vi "Lex Text-& UnescapedVariable-Text.vi"(8 "Error In":errorcluster) -> (0 "Error Out":errorcluster)   [LabVIEW 2018, in "Tests.lvlib" / "Lexer.lvlib"]
uses:
  Lexer.lvlib
  <vilib>/addons/_JKI Toolkits/Caraya/classes/Test/Test.lvclass
  <vilib>/addons/_JKI Toolkits/Caraya/classes/Assert/Assert.lvclass
  src/Toolkit/Low-Level/Tokens/Abstract/Abstract.lvclass
  src/Toolkit/Low-Level/Tokens/Text/Text.lvclass
  Tests.lvlib
  src/Toolkit/Low-Level/Tokens/UnescapedVariable/UnescapedVariable.lvclass
  D:/Users/cfield/Code/Field R&D Services/Mustache/trunk/src/Toolkit/Low-Level/Tokens/Abstract/Abstract.lvclass
  src/Toolkit/Toolkit.lvlib
  src/Toolkit/Low-Level/Support/Lex String.vi
  D:/Users/cfield/Code/Field R&D Services/Mustache/trunk/src/Toolkit/Low-Level/Tokens/Keyable/Keyable.lvclass
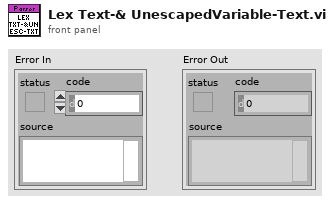
[diagram p1: front panel]
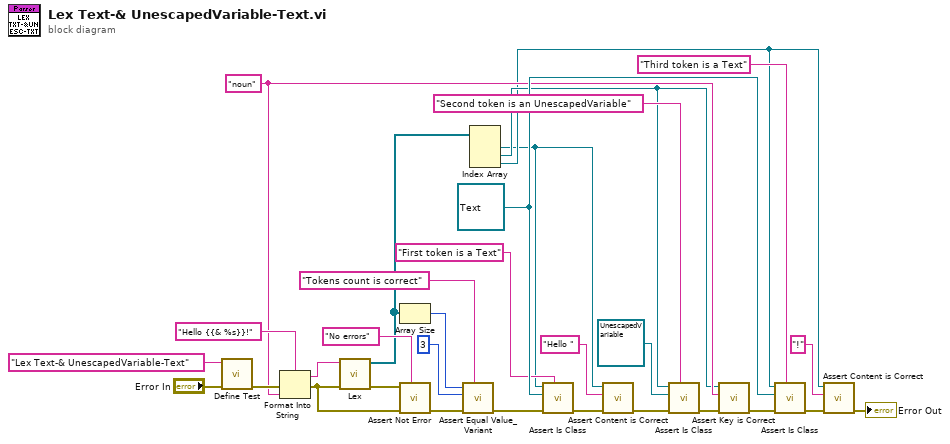
[diagram p0: block diagram]
diagram:
  w13 = refnum<class "Text.lvclass"> refnum ("Mustache.lvlib:Tokens.lvlib:Text.lvclass")
  w9 = "noun" ("String")
  n1 = call <vilib>:"Define Test.vi"("error in (no error)"="Error In", "Label (VI Title)"="Lex Text-& UnescapedVariable-Text") -> ("error out"=w28:errorcluster)  [unwired: 9 in]
  n2 = Format Into String(format string="Hello {{& %s}}!", error in=w28, w9) -> (resulting string=w1:string, error out=w2:errorcluster)  [unwired: 1 in]
  n3 = call-poly "Lex.vi"("Error In"=w2, "Input"=w1) -> ("Error Out"=w29:errorcluster, "Tokens"=w21:refnum<class "Abstract.lvclass">[])  [unwired: 8 in]
  n4 = Array Size(array=w21) -> (size(s)=w24:i32)
  n5 = call <vilib>:"Assert Not Error.vi"("Label"="No errors", "error in (no error)"=w2, "Not Error?"=w29) -> ("error out"=w26:errorcluster)  [unwired: 8 in]
  n6 = call <vilib>:"Assert Equal Value_Variant.vi"("Label"="Tokens count is correct", "error in (no error)"=w26, "Y"=3 ("size(s)"), "X"=w24) -> ("error out"=w22:errorcluster)  [unwired: 7 in]
  n7 = Index Array(array=w21) -> (element #1=w3:refnum<class "Abstract.lvclass">, element #2=w7:refnum<class "Abstract.lvclass">, element #3=w5:refnum<class "Abstract.lvclass">)  [unwired: 3 in]
  n8 = call "Assert Is Class.vi"("Label"="First token is a Text", "Error In"=w22, "Expected"=w13, "Actual"=w3) -> ("Error Out"=w19:errorcluster)  [unwired: 7 in]
  n9 = call "Assert Content is Correct.vi"("Error In"=w19, "Expected"="Hello ", "Token"=w3) -> ("Error Out"=w18:errorcluster)  [unwired: 8 in]
  n10 = call "Assert Is Class.vi"("Label"="Second token is an UnescapedVariable", "Error In"=w18, "Expected"=refnum<class "UnescapedVariable.lvclass"> refnum ("Mustache.lvlib:Tokens.lvlib:UnescapedVariable.lvclass"), "Actual"=w7) -> ("Error Out"=w8:errorcluster)  [unwired: 7 in]
  n11 = call "Assert Key is Correct.vi"("Error In"=w8, "Expected"=w9, "Token"=w7) -> ("Error Out"=w17:errorcluster)  [unwired: 8 in]
  n12 = call "Assert Is Class.vi"("Label"="Third token is a Text", "Error In"=w17, "Expected"=w13, "Actual"=w5) -> ("Error Out"=w16:errorcluster)  [unwired: 7 in]
  n13 = call "Assert Content is Correct.vi"("Error In"=w16, "Expected"="!", "Token"=w5) -> ("Error Out"=→"Error Out":errorcluster)  [unwired: 8 in]
